vi "Auton Kill Switch.vi"() -> ()   [LabVIEW 2017]
panel:
  in  "AutonKill?":bool
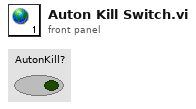
[diagram p1: front panel]
diagram:
